vi "Linux.Test.vi"() -> ()   [LabVIEW 2025]
uses:
  libzmq-v143-mt-4_3_6/LibZMQ.lvlib
panel:
  out "minor_ out":i32
  out "patch_ out":i32
  out "error out":errorcluster
  in  "error in (no error)":errorcluster
  out "major_ out":i32
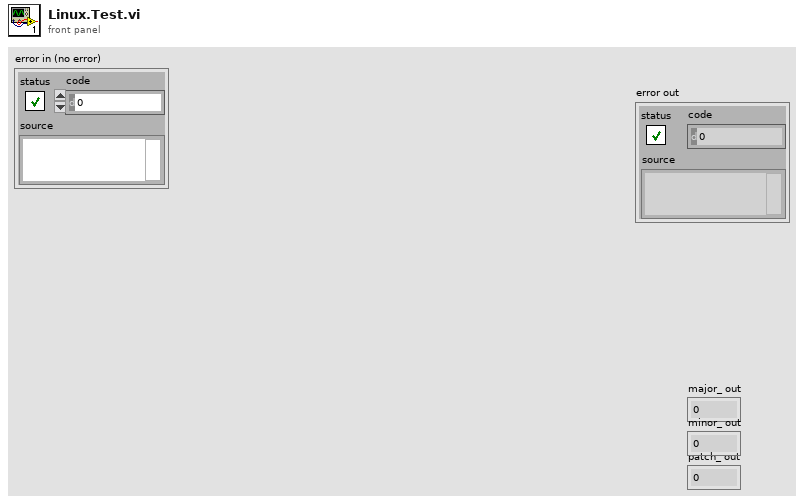
[diagram p1: front panel]
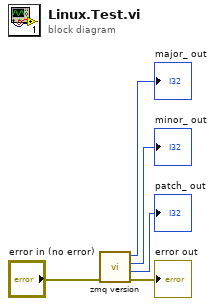
[diagram p0: block diagram]
diagram:
  n1 = call "zmq version.vi"("error in (no error)"="error in (no error)") -> ("error out"=→"error out":errorcluster, "patch_ out"=→"patch_ out":i32, "minor_ out"=→"minor_ out":i32, "major_ out"=→"major_ out":i32)  [unwired: 7 in]
